vi "old APU + 1 old Data Replay.vi"() -> ()   [LabVIEW 2015]
uses:
  <vilib>/Platform/TimedLoop/XDataNode/wakeup.ctl
  <vilib>/Platform/TimedLoop/XDataNode/XDNodeRunTimeDep.lvlib
  <vilib>/Platform/TimedLoop/XDataNode/nitl_modes.ctl
  <vilib>/Platform/TimedLoop/XDataNode/timing_clust.ctl
  <vilib>/Platform/TimedLoop/XDataNode/XDataNode.xnode
  <userlib>/_NI VeriStand FPGA Support/NI VeriStand RIO Library/Custom Device Components/Engine Simulation/Engine Simulation Globals.vi
  <vilib>/rvi/LocalResourceManager/LocalResourceManager.xnode
  <vilib>/rvi/DataTransferAndStorage/Container/XNode/niFpgaContainer.xnode
  <vilib>/eio/EIONode/EIONode.xnode
  <vilib>/rvi/eio/common/nirviEmuTemplateMethod_errors.vi
  <vilib>/rvi/DataTransferAndStorage/Container/Common/niFpgaContainerGetUniqueNameForEmu.vi
  <vilib>/rvi/DataTransferAndStorage/Container/Common/niFpgaContainerSetEmuInfo.vi
  <vilib>/rvi/eio/common/nirviEmuReportErrorAndStop.vi
  <vilib>/rvi/Memory/Memory_Emulation/niFpgaMemoryEmulationRefIn.vi
  <vilib>/rvi/Memory/Memory_Emulation/nirvimemoryEmulation.vi
  <vilib>/rvi/Memory/Memory_Emulation/nirvimemoryFastEmulation.vi
panel:
  in  "DataReplay.Data":i16[](array[numeric])=[0, 0, 0, 0, 0, 0, 0, 0, 0, 0, 0, 0, 0, 0, 0, 0, 0, 0, 0, 0, 0, 0, 0, 0, 0, 0, 0, 0, 0, 0, 0, 0]
  in  "DataReplay.LoadDone":bool
  in  "DataReplay.Select":i8
  in  "DataReplay.Toggle":bool
  in  "DataReplay.LoadOffset":u16
  in  "DataReplay.UpdateRate.<LOOP NAME>":u32=400
  in  "DataReplay.RPMThreshold.<LOOP NAME>.<REPLAY NAME>.<NUMBER>":u64
  in  "DataReplay.VScaleSlope.<LOOP NAME>.<REPLAY NAME>.<NUMBER>":u32
  in  "DataReplay.AngleToAddress.<LOOP NAME>.<REPLAY NAME>.<NUMBER>":u32
  in  "DataReplay.VScaleIntercept.<LOOP NAME>.<REPLAY NAME>.<NUMBER>":i32
  in  "DataReplay.CycleAngle?.<LOOP NAME>.<REPLAY NAME>.<NUMBER>":bool
  in  "DataReplay.ReverseNegate?.<LOOP NAME>.<REPLAY NAME>.<NUMBER>":bool
  in  "DataReplay.Offset.<LOOP NAME>.<REPLAY NAME>.<NUMBER>":u64
  in  "APU.Degrees per Tick":u64
  out "APU.Crank Angle":u64
  out "APU.Cycle Angle":u64
  in  "APU.Reset":bool
  in  "APU.Increment Rate":u64
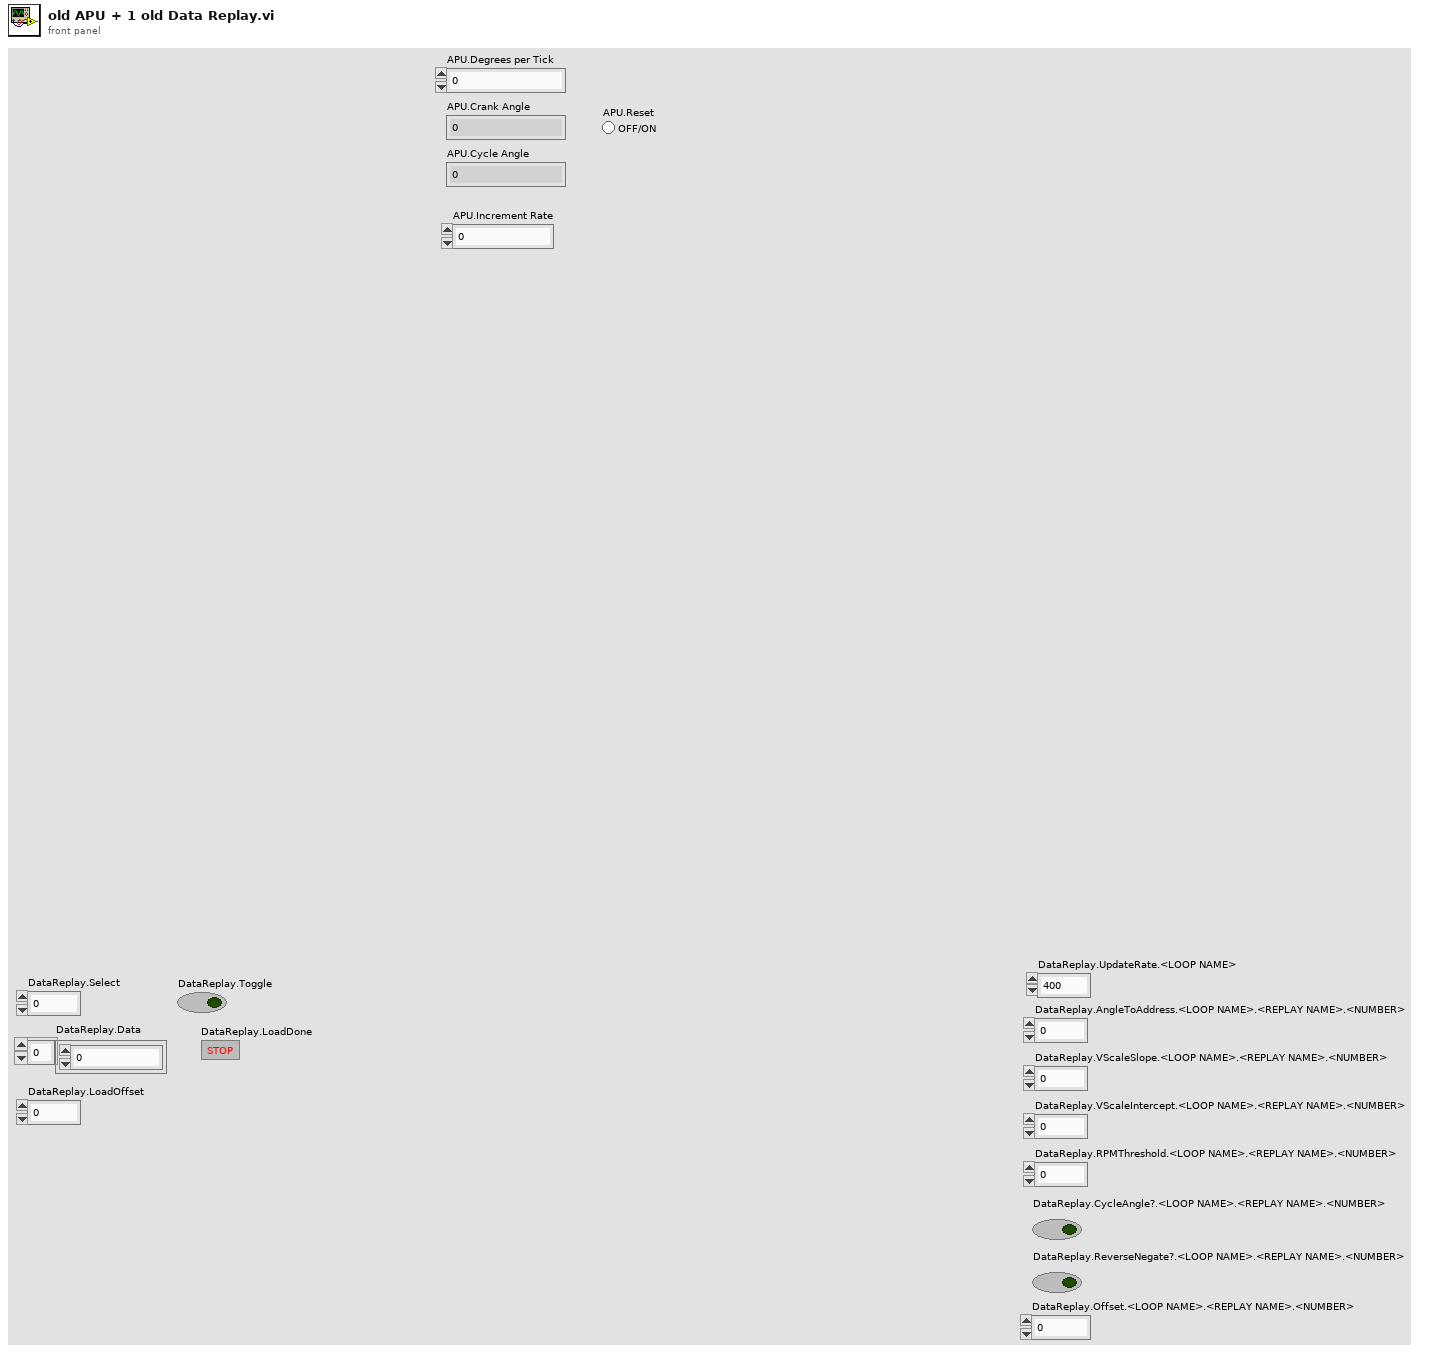
[diagram p1: front panel]
types:
  T1 = typedef "XDNodeRunTimeDep.lvlib/timing_clust.ctl" = cluster{"Expected End [f-1]":u64, "Actual End [f-1]":u64, "Finished Late? [f-1]":bool, "Expected End [i-1]":u64, "Actual End [i-1]":u64, "Finished Late? [i-1]":bool, "Expected Start [i]":u64, "Actual Start [i]":u64, "Expected Start [f]":u64, "Actual Start [f]":u64, "Source Name":string, "Structure Name":string, "Period":i64, "Deadline":i64, "Offset":i64, "Start":i64, "Priority":i32, "Timeout":i32, "Mode":T2, "Wakeup Reason":T3, "Error":errorcluster, "Source Type":string, "Secondary Source Type":string, "Global End Time":u64, "Global Start Time":u64, "Frame Duration":u64, "Iteration Duration":u64, "Assigned CPU":i32, "I/O Scan Engine Mode":u32}
  T2 = typedef "XDNodeRunTimeDep.lvlib/nitl_modes.ctl" = enum32{"No Change", "Process missed periods, maintain original phase", "Discard missed periods, maintain original phase", "Process missed periods, ignore original phase", "Discard missed periods, ignore original phase"}
  T3 = typedef "XDNodeRunTimeDep.lvlib/wakeup.ctl" = enum32{"Normal", "Aborted", "Asynchronous wakeup", "Timing source error", "Timed loop error", "Timeout"}
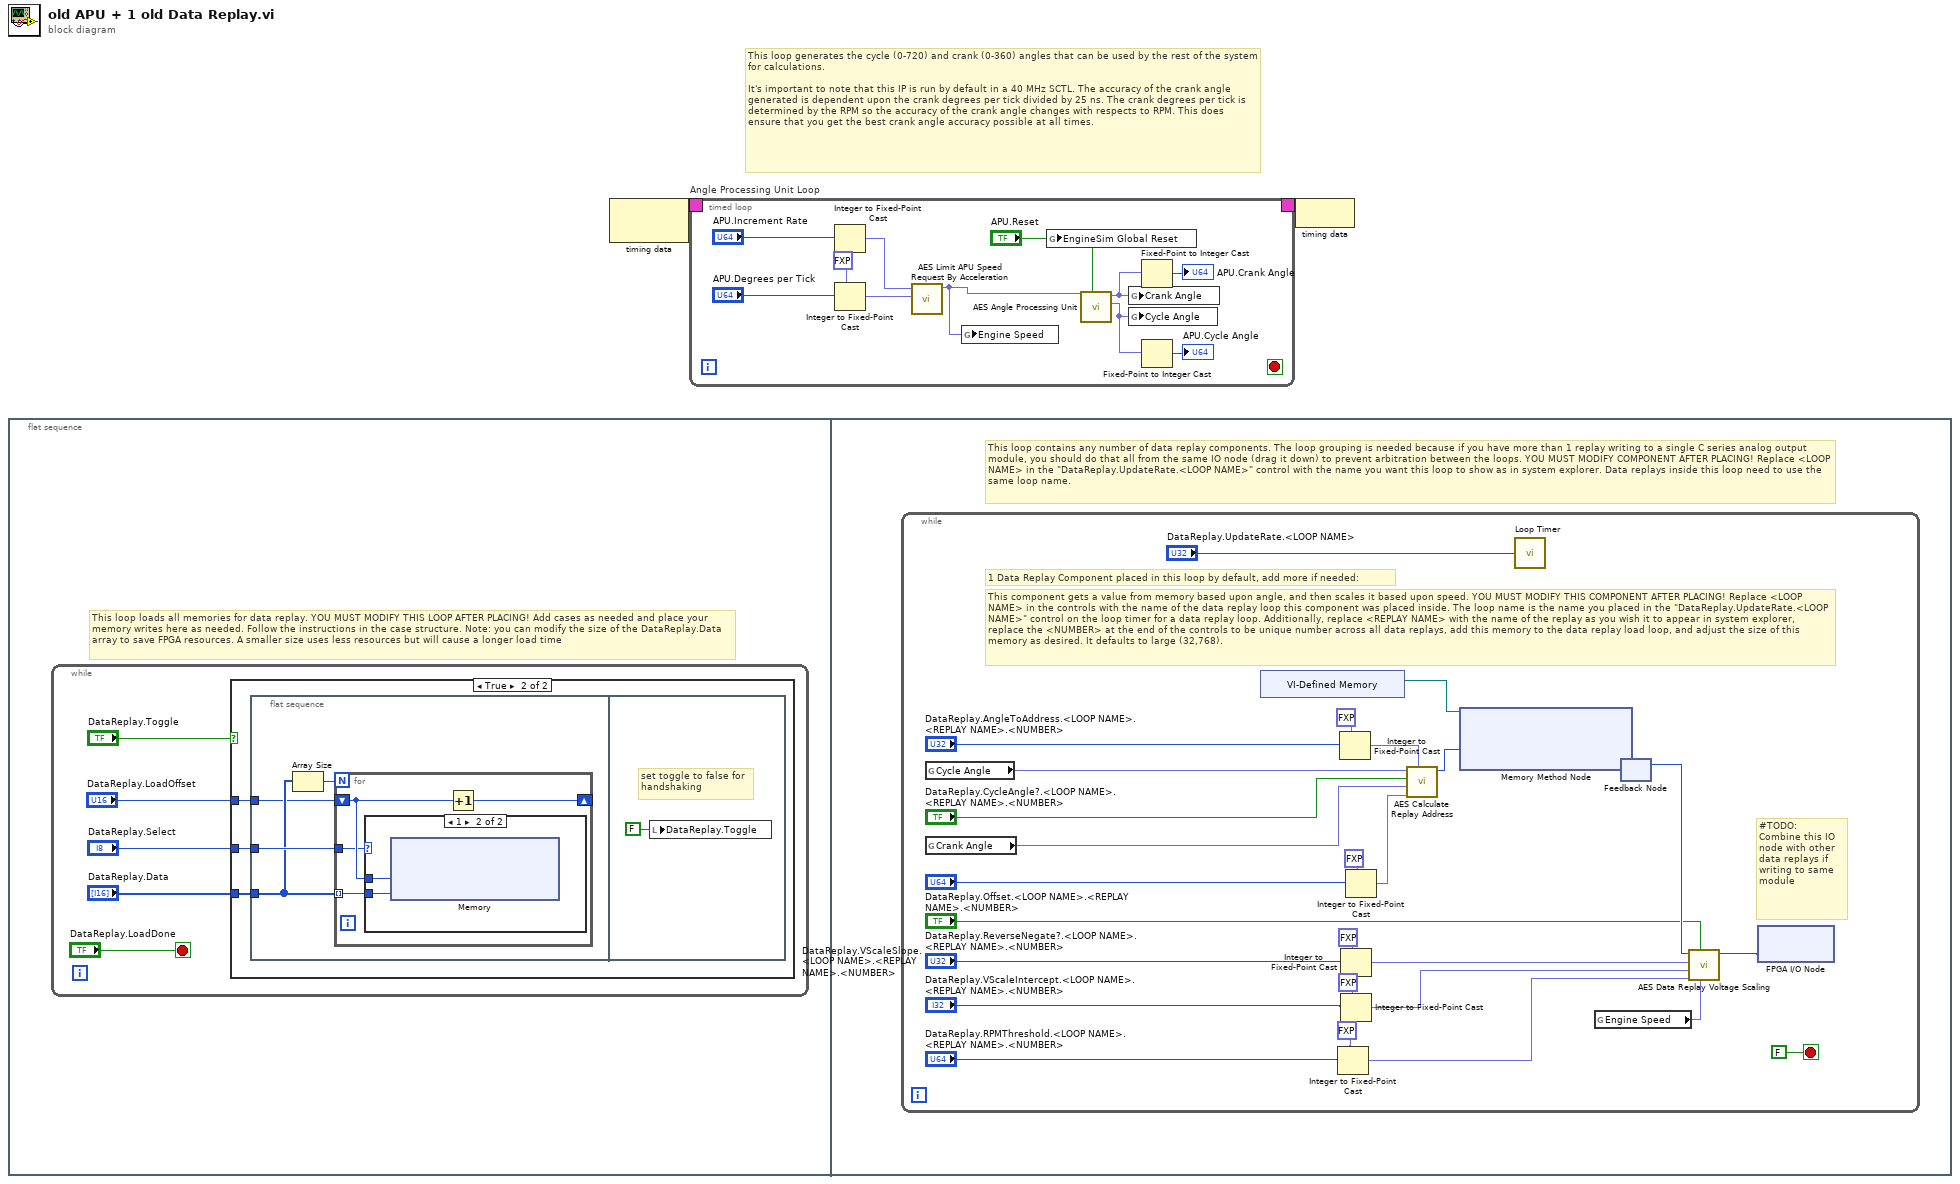
[diagram p0: block diagram]
diagram:
  # "This loop generates the cycle (0-720) and crank (0-360) angles that can be used by the rest of the system for calculations. \n\nIt's important to note that this IP is run by default in a 40 MHz SCTL. The accuracy of the crank angle generated is dependent upon the crank degrees per tick divided by 25 ns. The crank degrees per tick is determined by the RPM so the accuracy of the crank angle changes with respects to RPM. This does ensure that you get the best crank angle accuracy possible at all times."
  n1 = flat-sequence {
    frame #0 {
      # "This loop loads all memories for data replay. YOU MUST MODIFY THIS LOOP AFTER PLACING! Add cases as needed and place your memory writes here as needed. Follow the instructions in the case structure. Note: you can modify the size of the DataReplay.Data array to save FPGA resources. A smaller size uses less resources but will cause a longer load time"
      n2 = while {
        stop <- "DataReplay.LoadDone" stop-if-true
        n3 = case shown="True" "DataReplay.Toggle" {
          tunnel: "DataReplay.Data" -> [_ w10]
          tunnel: "DataReplay.Select" -> [_ w9]
          tunnel: "DataReplay.LoadOffset" -> [_ w8]
          frame False {
          }
          frame True {
            n4 = flat-sequence {
              tunnel: w10 -> [w13]
              tunnel: w9 -> [w14]
              tunnel: w8 -> [w11]
              frame #0 {
                n5 = Array Size(array=w13) -> (size(s)=w12:i32)
                n6 = for {
                  N: w12 -> [_]
                  tunnel: w13 -> [w18] mode=indexing
                  shift-right: [w17] -> _
                  shift-left: w11 -> [w16]
                  tunnel: w14 -> [w15]
                  n7 = case shown="1" w15 {
                    tunnel: w18 -> [_ w19]
                    tunnel: w16 -> [_ w20]
                    frame Default {
                      # "leave this blank"
                    }
                    frame 1 {
                      n8 = xnode "Memory"("Address"=w20, "Data"=w19) -> ()  [unwired: 1 in, 1 out]
                    }
                  }
                  n9 = Increment(x=w16) -> (x+1=w17:u16)
                }
              }
              frame #1 {
                # "set toggle to false for\nhandshaking"
                n10 = local write "DataReplay.Toggle"(FALSE ("DataReplay.Toggle")) -> ()
              }
            }
          }
        }
      }
    }
    frame #1 {
      # "This loop contains any number of data replay components. The loop grouping is needed because if you have more than 1 replay writing to a single C series analog output module, you should do that all from the same IO node (drag it down) to prevent arbitration between the loops. YOU MUST MODIFY COMPONENT AFTER PLACING! Replace <LOOP NAME> in the \"DataReplay.UpdateRate.<LOOP NAME>\" control with the name you want this loop to show as in system explorer. Data replays inside this loop need to use the same loop name."
      n11 = while {
        stop <- FALSE stop-if-true
        # "#TODO:\nCombine this IO node with other data replays if writing to same module"
        # "This component gets a value from memory based upon angle, and then scales it based upon speed. YOU MUST MODIFY THIS COMPONENT AFTER PLACING! Replace <LOOP NAME> in the controls with the name of the data replay loop this component was placed inside. The loop name is the name you placed in the \"DataReplay.UpdateRate.<LOOP NAME>\" control on the loop timer for a data replay loop. Additionally, replace <REPLAY NAME> with the name of the replay as you wish it to appear in system explorer, replace the <NUMBER> at the end of the controls to be unique number across all data replays, add this memory to the data replay load loop, and adjust the size of this memory as desired. It defaults to large (32,768)."
        # "1 Data Replay Component placed in this loop by default, add more if needed:"
        n12 = global read "Engine Simulation Globals.vi" "Cycle Angle"() -> (w28:fxp<+,61,10>)
        n13 = global read "Engine Simulation Globals.vi" "Crank Angle"() -> (w26:fxp<+,60,9>)
        n14 = xnode "VI-Defined Memory"() -> ("Memory Out"=w38:refnum<k21>)
        n15 = Integer to Fixed-Point Cast(fixed-point type=fxp<+/-,47,-4> 0.0 ("Crank.Degrees per Tick"), integer="DataReplay.RPMThreshold.<LOOP NAME>.<REPLAY NAME>.<NUMBER>") -> (fixed-point=w32:fxp<+/-,47,-4>)
        n16 = Integer to Fixed-Point Cast(fixed-point type=fxp<+,18,7> 0.0 ("Crank.Degrees per Tick"), integer="DataReplay.AngleToAddress.<LOOP NAME>.<REPLAY NAME>.<NUMBER>") -> (fixed-point=w29:fxp<+,18,7>)
        n17 = Integer to Fixed-Point Cast(fixed-point type=fxp<+,18,12> 0.0 ("Crank.Degrees per Tick"), integer="DataReplay.VScaleSlope.<LOOP NAME>.<REPLAY NAME>.<NUMBER>") -> (fixed-point=w34:fxp<+,18,12>)
        n18 = Integer to Fixed-Point Cast(fixed-point type=fxp<+/-,18,3> 0.0 ("Crank.Degrees per Tick"), integer="DataReplay.VScaleIntercept.<LOOP NAME>.<REPLAY NAME>.<NUMBER>") -> (fixed-point=w33:fxp<+/-,18,3>)
        n19 = Integer to Fixed-Point Cast(fixed-point type=fxp<+/-,61,10> 0.0 ("FullyCustomTeeth.Cams.Cam1.Offset"), integer="DataReplay.Offset.<LOOP NAME>.<REPLAY NAME>.<NUMBER>") -> (fixed-point=w23:fxp<+/-,61,10>)
        n20 = call <userlib>:"AES Calculate Replay Address.vi"("AngleToAddress"=w29, "Offset (0)"=w23, "Crank Angle"=w26, "CycleAngle?"="DataReplay.CycleAngle?.<LOOP NAME>.<REPLAY NAME>.<NUMBER>", "Cycle Angle"=w28) -> ("memory address"=w30:u32)  [unwired: 6 in]
        n21 = xnode ("Memory Method Node")("Address"=w30, "Memory In"=w38) -> ("Data"=w37:i16)  [unwired: 1 out]
        n22 = call "Loop Timer"("Count(Ticks)"="DataReplay.UpdateRate.<LOOP NAME>") -> ()  [unwired: 1 out]
        n23 = global read "Engine Simulation Globals.vi" "Engine Speed"() -> (w35:fxp<+/-,47,-4>)
        n24 = feedback #1() -> (w36:i16)  [unwired: 1 in]
        n25 = feedback-in #1(w37) -> ()
        n26 = call <userlib>:"AES Data Replay Voltage Scaling.vi"("APU.Degrees per Tick"=w35, "negate voltage when speed negative?"="DataReplay.ReverseNegate?.<LOOP NAME>.<REPLAY NAME>.<NUMBER>", "speed threshold"=w32, "voltage scaling intercept"=w33, "voltage scaling slope"=w34, "replay data"=w36) -> ("output value"=w22:i16)  [unwired: 5 in]
        n27 = xnode "FPGA I/O Node"("AO0"=w22) -> ()  [unwired: 1 in, 1 out]
      }
    }
  }
  n28 = node-c288() -> (w2:T1)  [unwired: 1 in]
  n29 = timed-loop "Angle Processing Unit Loop" {
    timing: w2 -> [_]
    timing-out: [_] -> w1
    stop <- _ stop-if-true
    w51 = fxp<+/-,47,-4> 0.0 ("Crank.Degrees per Tick")
    n30 = Integer to Fixed-Point Cast(fixed-point type=w51, integer="APU.Increment Rate") -> (fixed-point=w50:fxp<+/-,47,-4>)
    n31 = Integer to Fixed-Point Cast(fixed-point type=w51, integer="APU.Degrees per Tick") -> (fixed-point=w53:fxp<+/-,47,-4>)
    n32 = call <userlib>:"AES Limit APU Speed Request By Acceleration.vi"("APU.Degrees per Tick in"=w53, "APU.Increment Rate"=w50) -> ("APU.Degrees per Tick out"=w49:fxp<+/-,47,-4>)  [unwired: 9 in]
    n33 = global write "Engine Simulation Globals.vi" "Engine Speed"(w49) -> ()
    n34 = global write "Engine Simulation Globals.vi" "EngineSim Global Reset"("APU.Reset") -> ()
    n35 = call <userlib>:"AES Angle Processing Unit.vi"("APU.Reset"="APU.Reset", "APU.Degrees per Tick"=w49) -> ("APU.Cycle Angle"=w55:fxp<+,61,10>, "APU.Crank Angle"=w59:fxp<+,60,9>)  [unwired: 8 in]
    n36 = global write "Engine Simulation Globals.vi" "Crank Angle"(w59) -> ()
    n37 = global write "Engine Simulation Globals.vi" "Cycle Angle"(w55) -> ()
    n38 = Fixed-Point to Integer Cast(1:w59) -> (0:→"APU.Crank Angle":u64)
    n39 = Fixed-Point to Integer Cast(1:w55) -> (0:→"APU.Cycle Angle":u64)
  }
  n40 = node-c288(w1) -> ()
